vi "GetSetDeviation.vi"(7 "Deviation value":dbl min=0.0 max=25.0 step=1.0, 8 "error in":errorcluster, 9 "Channel Number (1-4)":T1=1 items=["Channel 1"=1, "Channel 2"=2, "Channel 3"=3, "Channel 4"=4], 10 "get/set":T2=enum."set", 11 "VISA resource name":refnum<visa-resource-name>) -> (0 "error out":errorcluster, 2 "Deviation":string, 3 "VISA resource name out":refnum<visa-resource-name>)   [LabVIEW 2023, in "Thermotron 8800.lvlib"]
doc: "DEVN\nCommand name: Send deviation reading or load deviation setting\nCommand type: Variable; edit from hold\nDescription: The query command asks the 8800 for the current deviation reading from a selected\nchannel. The 8800 sends the value in the channel’s selected units. The operation\ncommand loads a deviation setting into the 8800 for the current manual mode\noperation, or sends a temporary deviation value during an edit from hold operation.\nSyntax: DEVNn? or DEVNn,data\nWhere n is any control channel (1 through 4).\nData type: Decimal\nQuery example: DEVN1?\n8800 response: 2.3 (The current deviation reading for control channel 1 is 2.3.)\nOperation example: DEVN2,5\n8800 response: 0 (If the 8800 is in manual mode, it loads a deviation value of 5 units into control\nchannel 2.)"
uses:
  Thermotron 8800.lvlib
  Private/get set.ctl
  Private/AnalogInputChannelNumber 1-4.ctl
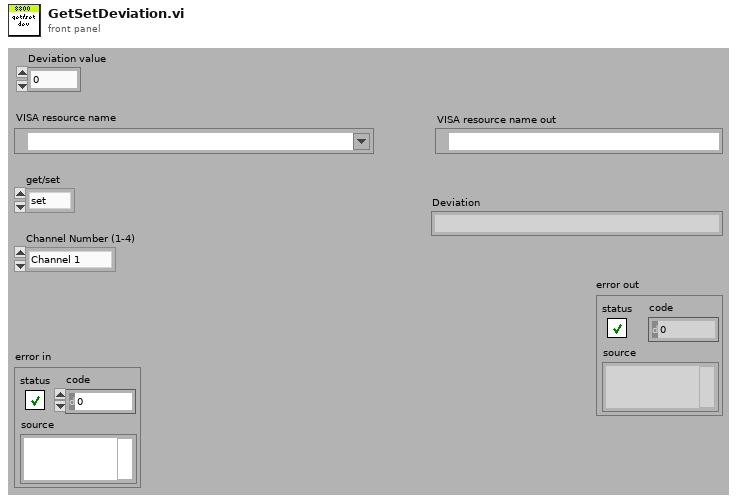
[diagram p1: front panel]
types:
  T1 = typedef "Thermotron 8800.lvlib/AnalogInputChannelNumber 1-4.ctl" = u16
  T2 = typedef "Thermotron 8800.lvlib/get set.ctl" = enum16{"get", "set"}
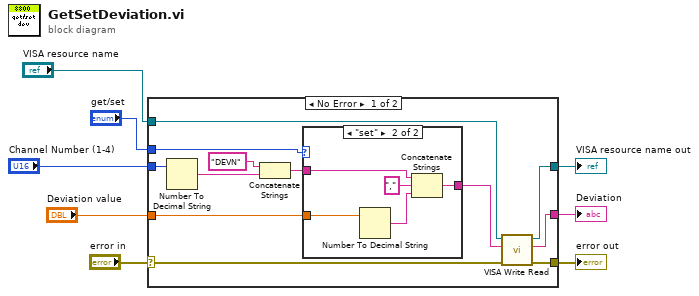
[diagram p0: block diagram]
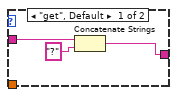
[diagram p2: hidden frame]
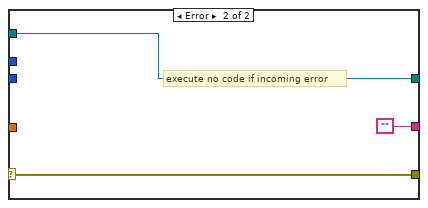
[diagram p3: hidden frame]
diagram:
  n1 = case shown="No Error" "error in" {
    selector: "error in" -> [w10 w31]
    tunnel: [w19 w31] -> w8
    tunnel: [w18 w30] -> w7
    tunnel: "VISA resource name" -> [w17 w30]
    tunnel: "Channel Number (1-4)" -> [w15 _]
    tunnel: "get/set" -> [w12 _]
    tunnel: [w11 ""] -> w3
    tunnel: "Deviation value" -> [w9 _]
    frame No Error {
      n2 = Number To Decimal String(number=w15) -> (decimal integer string=w14:string)  [unwired: 1 in]
      n3 = Concatenate Strings("DEVN" ("8800 Command"), w14) -> (w13:string)
      n4 = case shown="\"set\"" w12 {
        tunnel: w13 -> [w22 w28]
        tunnel: [w23 w25] -> w20
        tunnel: w9 -> [_ w24]
        frame "get", Default {
          n5 = Concatenate Strings(w22, "?" ("8800 Command")) -> (w23:string)
        }
        frame "set" {
          n6 = Number To Decimal String(number=w24) -> (decimal integer string=w26:string)  [unwired: 1 in]
          n7 = Concatenate Strings(w28, "," ("string"), w26) -> (w25:string)
        }
      }
      n8 = call "VISA Write Read.vi"("error in (no error)"=w10, "8800 Command"=w20, "VISA Refnum in"=w17) -> ("error out"=w19:errorcluster, "read buffer"=w11:string, "VISA Refnum out"=w18:refnum<visa-resource-name>)  [unwired: 6 in]
    }
    frame Error {
      # "execute no code if incoming error"
    }
  }
  "VISA resource name out" <- w7
  "error out" <- w8
  "Deviation" <- w3
